vi "Finish.vi"   [LabVIEW 2014]
doc: "This VI is called just before exiting. It is expected to close I/O refnum, save collected data, etc."
uses:
  <vilib>/Rock Robotics/WPI/Joystick/WPI_JoystickGetSetRefNum.vi
  <vilib>/Rock Robotics/WPI/RobotDrive/WPI_RobotDriveGetSetRefNum.vi
  Robot Global Data.vi
  SimpleGyro/SimpleGyro.lvlib
types:
  T1 = typedef "WPI_EncoderDevRef.ctl" = cluster{"DevStatus":errorcluster, "EncoderIndex":T2, "CounterIndex":T3, "DistancePerCount":dbl, "Decoding Type":T4}
  T2 = typedef "FPGA_EncoderIdx.ctl" = enum8{"Enc 0", "Enc 1", "Enc 2", "Enc 3", "Enc 4", "Enc 5", "Enc 6", "Enc 7", "Invalid"}
  T3 = typedef "FPGA_CounterCtrSystemIndex.ctl" = enum8{"Ctr 0", "Ctr 1", "Ctr 2", "Ctr 3", "Ctr 4", "Ctr 5", "Ctr 6", "Ctr 7", "Invalid"}
  T4 = typedef "WPI_EncoderType.ctl" = enum16{"1x", "2x", "4x"}
  T5 = typedef "WPI_I2CDevRef.ctl" = cluster{"DevStatus":errorcluster, "Controller":T6, "Device Address":u8, "Handle":i32, "I2C Bus":T7}
  T6 = typedef "FPGA_TypedefDigitalModule.ctl" = enum16{"Controller 1"}
  T7 = typedef "i2c_bus.ctl" = enum16{"I2C On-Board", "I2C MXP", "Invalid"}
  T8 = typedef "WPI_RelayDevRef.ctl" = cluster{"DevStatus":errorcluster, "Relay Channel":T9, "Controller":T6, "Relay Direction":T10}
  T9 = typedef "FPGA_DIORelayChannel.ctl" = enum8{"Relay 0", "Relay 1", "Relay 2", "Relay 3", "Invalid"}
  T10 = typedef "WPI_RelayDirection.ctl" = enum16{"Both directions", "Forward only", "Reverse only"}
  T11 = typedef "WPI_JoystickDevRef.ctl" = cluster{"Device":T12}
  T12 = typedef "WPI_JoystickDeviceEnum.ctl" = enum16{"USB 0", "USB 1", "USB 2", "USB 3", "USB 4", "USB 5"}
  T13 = typedef "WPI_RobotDriveDevRef.ctl" = cluster{"DevStatus":errorcluster, "Motors[]":T14[], "Square Inputs":bool, "Max Output":dbl}
  T14 = typedef "WPI_MotorControlDeviceRef.ctl" = cluster{"DeviceStatus":errorcluster, "Type":T15, "PWM":cluster{"Controller":T6, "PWM Channel":T16, "DeadBand":T17}, "CAN":cluster{"Device Number":u8, "Control Mode":T18, "Semaphore":T19, "Max Vout":dbl, "TalonSRX Control Mode":T20}, "Invert":bool, "TransformRef":T21, "InvTransformRef":T21}
  T15 = typedef "WPI_MotorControlType.ctl" = enum16{"PWM", "CAN", "CANTalonSRX"}
  T16 = typedef "FPGA_DIOPWMChannel.ctl" = enum8{"PWM 0", "PWM 1", "PWM 2", "PWM 3", "PWM 4", "PWM 5", "PWM 6", "PWM 7", "PWM 8", "PWM 9", "PWM MXP 0", "PWM MXP 1", "PWM MXP 2", "PWM MXP 3", "PWM MXP 4", "PWM MXP 5", "PWM MXP 6", "PWM MXP 7", "PWM MXP 8", "PWM MXP 9", "Invalid"}
  T17 = typedef "WPI_PWMDeadband.ctl" = cluster{"Name":string, "maxPositivePwm":i32, "minPositivePwm":i32, "centerPwm":i32, "maxNegativePwm":i32, "minNegativePwm":i32, "angularRange":u16}
  T18 = typedef "WPI_CANJaguar_ControlMode.ctl" = enum8{"Percent VBus", "Current", "Speed", "Position", "Voltage"}
  T19 = typedef "Semaphore RefNum" = refnum<k1>
  T20 = typedef "WPI_CANTalonSRX_APIControlMode.ctl" = enum8{"Percent VBus", "Speed", "Position", "Slave", "Unchanged / Invalid"}
  T21 = typedef "WPI_PWMTransform_ConPane.ctl" = refnum<vi>
  T22 = typedef "SimpleGyro.lvlib/WPI_SimpleGyroDevRef.ctl" = cluster{"DevStatus":errorcluster, "Handle":i32, "Controller":T6, "SPI Bus":T23, "Device Found":bool, "Sample Rate":dbl}
  T23 = typedef "spi_bus.ctl" = enum16{"SPI On-Board, CS0", "SPI On-Board, CS1", "SPI On-Board, CS2", "SPI On-Board, CS3", "SPI MXP", "Invalid"}
  T24 = typedef "WPI_SwitchDevRef.ctl" = cluster{"DevStatus":errorcluster, "DIO Channel":T25, "Controller":T6, "CntIndex":T3, "Normally Closed":bool}
  T25 = typedef "FPGA_DIOChannel.ctl" = enum8{"DIO 0", "DIO 1", "DIO 2", "DIO 3", "DIO 4", "DIO 5", "DIO 6", "DIO 7", "DIO 8", "DIO 9", "DIO MXP 0", "DIO MXP 1", "DIO MXP 2", "DIO MXP 3", "DIO MXP 4", "DIO MXP 5", "DIO MXP 6", "DIO MXP 7", "DIO MXP 8", "DIO MXP 9", "DIO MXP 10", "DIO MXP 11", "DIO MXP 12", "DIO MXP 13", "DIO MXP 14", "DIO MXP 15", "Invalid"}
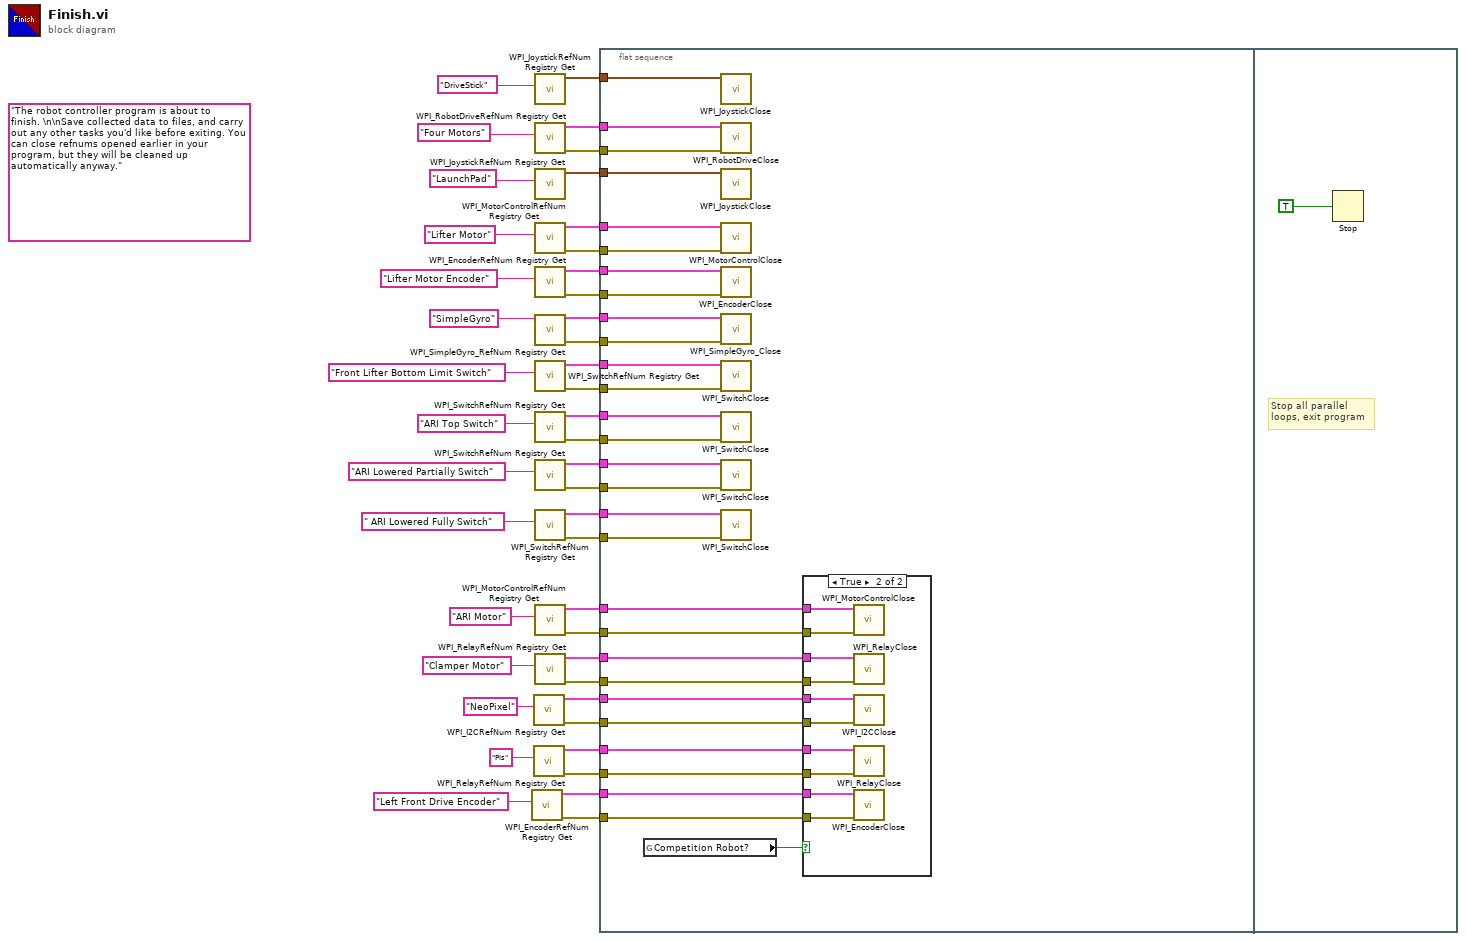
[diagram p0: block diagram]
diagram:
  (unwired) "The robot controller program is about to finish. \n\nSave collected data to files, and carry out any other tasks you'd like before exiting. You can close refnums opened earlier in your program, but they will be cleaned up automatically anyway."
  n1 = call <vilib>:"WPI_EncoderRefNum Registry Get.vi"("refnum name"="Left Front Drive Encoder") -> ("error out"=w4:errorcluster, "EncoderDevRef"=w5:T1)  [unwired: 9 in]
  n2 = call <vilib>:"WPI_I2CRefNum Registry Get.vi"("refnum name"="NeoPixel") -> ("error out"=w8:errorcluster, "I2CDevRef"=w9:T5)  [unwired: 9 in]
  n3 = call <vilib>:"WPI_RelayRefNum Registry Get.vi"("refnum name"="PIs") -> ("error out"=w6:errorcluster, "RelayDevRef"=w7:T8)  [unwired: 9 in]
  n4 = call <vilib>:"WPI_JoystickRefNum Registry Get.vi"("refnum name"="DriveStick") -> ("JoystickDevRef"=w40:T11)  [unwired: 1 in, 9 out]
  n5 = call <vilib>:"WPI_RobotDriveRefNum Registry Get.vi"("refnum name"="Four Motors") -> ("error out"=w39:errorcluster, "RobotDriveDevRef"=w41:T13)  [unwired: 1 in, 8 out]
  n6 = call <vilib>:"WPI_JoystickRefNum Registry Get.vi"("refnum name"="LaunchPad") -> ("JoystickDevRef"=w37:T11)  [unwired: 1 in, 9 out]
  n7 = call <vilib>:"WPI_MotorControlRefNum Registry Get.vi"("refnum name"="Lifter Motor") -> ("error out"=w29:errorcluster, "MotorControlDevRef"=w30:T14)  [unwired: 9 in]
  n8 = call <vilib>:"WPI_EncoderRefNum Registry Get.vi"("refnum name"="Lifter Motor Encoder") -> ("error out"=w27:errorcluster, "EncoderDevRef"=w28:T1)  [unwired: 9 in]
  n9 = call "WPI_SimpleGyro_RefNum Registry Get.vi"("refnum name"="SimpleGyro") -> ("error out"=w1:errorcluster, "SimpleGyroDevRef"=w3:T22)  [unwired: 9 in]
  n10 = call <vilib>:"WPI_SwitchRefNum Registry Get.vi"("refnum name"="Front Lifter Bottom Limit Switch") -> ("error out"=w25:errorcluster, "SwitchDevRef"=w26:T24)  [unwired: 9 in]
  n11 = call <vilib>:"WPI_SwitchRefNum Registry Get.vi"("refnum name"="ARI Top Switch") -> ("error out"=w23:errorcluster, "SwitchDevRef"=w24:T24)  [unwired: 9 in]
  n12 = call <vilib>:"WPI_SwitchRefNum Registry Get.vi"("refnum name"="ARI Lowered Partially Switch") -> ("error out"=w21:errorcluster, "SwitchDevRef"=w22:T24)  [unwired: 9 in]
  n13 = call <vilib>:"WPI_SwitchRefNum Registry Get.vi"("refnum name"=" ARI Lowered Fully Switch") -> ("error out"=w19:errorcluster, "SwitchDevRef"=w20:T24)  [unwired: 9 in]
  n14 = call <vilib>:"WPI_MotorControlRefNum Registry Get.vi"("refnum name"="ARI Motor") -> ("error out"=w12:errorcluster, "MotorControlDevRef"=w13:T14)  [unwired: 9 in]
  n15 = call <vilib>:"WPI_RelayRefNum Registry Get.vi"("refnum name"="Clamper Motor") -> ("error out"=w10:errorcluster, "RelayDevRef"=w11:T8)  [unwired: 9 in]
  n16 = flat-sequence {
    tunnel: w41 -> [w72]
    tunnel: w40 -> [w71]
    tunnel: w39 -> [w70]
    tunnel: w37 -> [w69]
    tunnel: w30 -> [w68]
    tunnel: w29 -> [w67]
    tunnel: w28 -> [w66]
    tunnel: w27 -> [w65]
    tunnel: w26 -> [w64]
    tunnel: w25 -> [w63]
    tunnel: w24 -> [w62]
    tunnel: w23 -> [w61]
    tunnel: w22 -> [w60]
    tunnel: w21 -> [w59]
    tunnel: w20 -> [w58]
    tunnel: w19 -> [w57]
    tunnel: w13 -> [w56]
    tunnel: w12 -> [w55]
    tunnel: w11 -> [w54]
    tunnel: w10 -> [w53]
    tunnel: w9 -> [w52]
    tunnel: w8 -> [w51]
    tunnel: w7 -> [w50]
    tunnel: w6 -> [w49]
    tunnel: w5 -> [w48]
    tunnel: w4 -> [w47]
    tunnel: w3 -> [w46]
    tunnel: w1 -> [w45]
    frame #0 {
      n17 = global read "Robot Global Data.vi" "Competition Robot?"() -> (w44:bool)
      n18 = call <vilib>:"WPI_JoystickClose.vi"("JoystickDevRef"=w71) -> ()  [unwired: 11 out]
      n19 = call <vilib>:"WPI_RobotDriveClose.vi"("error in (no error)"=w70, "RobotDriveDevRef"=w72) -> ()  [unwired: 10 out]
      n20 = call <vilib>:"WPI_JoystickClose.vi"("JoystickDevRef"=w69) -> ()  [unwired: 11 out]
      n21 = call <vilib>:"WPI_MotorControlClose.vi"("error in (no error)"=w67, "MotorControlDevRef"=w68) -> ()  [unwired: 9 in, 1 out]
      n22 = call <vilib>:"WPI_EncoderClose.vi"("error in (no error)"=w65, "EncoderDevRef"=w66) -> ()  [unwired: 9 in, 1 out]
      n23 = call "WPI_SimpleGyro_Close.vi"("error in"=w45, "SimpleGyroDevRef"=w46) -> ()  [unwired: 9 in, 1 out]
      n24 = call <vilib>:"WPI_SwitchClose.vi"("error in (no error)"=w63, "SwitchDevRef"=w64) -> ()  [unwired: 9 in, 1 out]
      n25 = call <vilib>:"WPI_SwitchClose.vi"("error in (no error)"=w61, "SwitchDevRef"=w62) -> ()  [unwired: 9 in, 1 out]
      n26 = call <vilib>:"WPI_SwitchClose.vi"("error in (no error)"=w59, "SwitchDevRef"=w60) -> ()  [unwired: 9 in, 1 out]
      n27 = call <vilib>:"WPI_SwitchClose.vi"("error in (no error)"=w57, "SwitchDevRef"=w58) -> ()  [unwired: 9 in, 1 out]
      n28 = case shown="True" w44 {
        tunnel: w56 -> [_ w82]
        tunnel: w55 -> [_ w81]
        tunnel: w54 -> [_ w80]
        tunnel: w53 -> [_ w79]
        tunnel: w52 -> [_ w78]
        tunnel: w51 -> [_ w77]
        tunnel: w50 -> [_ w76]
        tunnel: w49 -> [_ w75]
        tunnel: w48 -> [_ w74]
        tunnel: w47 -> [_ w73]
        frame False {
        }
        frame True {
          n29 = call <vilib>:"WPI_MotorControlClose.vi"("error in (no error)"=w81, "MotorControlDevRef"=w82) -> ()  [unwired: 9 in, 1 out]
          n30 = call <vilib>:"WPI_RelayClose.vi"("error in (no error)"=w79, "RelayDevRef"=w80) -> ()  [unwired: 9 in, 1 out]
          n31 = call <vilib>:"WPI_I2CClose.vi"("error in (no error)"=w77, "I2CDevRef"=w78) -> ()  [unwired: 9 in, 1 out]
          n32 = call <vilib>:"WPI_RelayClose.vi"("error in (no error)"=w75, "RelayDevRef"=w76) -> ()  [unwired: 9 in, 1 out]
          n33 = call <vilib>:"WPI_EncoderClose.vi"("error in (no error)"=w73, "EncoderDevRef"=w74) -> ()  [unwired: 9 in, 1 out]
        }
      }
    }
    frame #1 {
      # "Stop all parallel\nloops, exit program"
      n34 = Stop(stop? (T)=TRUE ("Quit")) -> ()
    }
  }
